vi "setpoints.vi"(6 "error in (no error)":errorcluster, 7 "setpoints":T2={"graph data interval (s)"=5.0, "sludge flow [L/s]"=0.001, "plant flow [L/s]"=0.5, "Plant Flow PID "={"proportional gain (Kc)"=10.0, "integral time (Ti, min)"=0.4, "derivative time (Td, min)"=0.0}, "Sludge PID "={"proportional gain (Kc)"=0.07, "integral time (Ti, min)"=1.0, "derivative time (Td, min)"=0.01}, "backwash"={"Filtered quality target [NTU]"=0.2, "min filtration time [s]"=3600.0, "Ripen time [s]"=600.0}, "Coagulant"={"flocculator volume (L)"=66.81, "clarifier volume (L)"=2.0, "dose updates per HRT"=10, "target clarified turbidity (NTU)"=0.6, "Coagulant mode"=enum."manual", "Coag dose [mg/L]"=5.5, "pump mL/rev"=0.255, "clarifier flow [L/s]"=0.0033, "min Coag dose [mg/L]"=2.0, "max Coag dose [mg/L]"=6.0, "Steps"=3, "HRT response delay"=2, "Ku*"=1.0, "DOM coag demand [mg/L]"=0.0, "min DOM coag demand [mg/L]"=0.0, "max DOM coag demand [mg/L]"=0.0}} {"Coagulant"."max DOM coag demand [mg/L]" min=0.0 max=20.0 step=0.1; "Coagulant"."min DOM coag demand [mg/L]" min=0.0 max=10.0 step=0.1; "Coagulant"."DOM coag demand [mg/L]" min=0.0 max=20.0 step=0.1; "Coagulant"."HRT response delay" min=1 max=10 step=1; "Coagulant"."Steps" min=3 step=1; "Coagulant"."clarifier flow [L/s]" min=0.0001 max=1.0 step=0.0001; "Coagulant"."target clarified turbidity (NTU)" min=0.1 max=5.0 step=0.01; "Coagulant"."dose updates per HRT" min=1 max=100 step=1; "Sludge PID"."derivative time (Td, min)" format="%.3f"; "Sludge PID"."integral time (Ti, min)" format="%.3f"; "Sludge PID"."proportional gain (Kc)" format="%.3f"; "Plant Flow PID"."derivative time (Td, min)" format="%.3f"; "Plant Flow PID"."integral time (Ti, min)" format="%.3f"; "Plant Flow PID"."proportional gain (Kc)" format="%.3f"; "plant flow [L/s]" min=0.05 max=1.0 step=0.05; "sludge flow [L/s]" min=0.0 max=0.05 step=0.001; "graph data interval (s)" min=1 max=1000 step=1}, 9 "ini":T1) -> (4 "error out":errorcluster, 5 "Setpoints out":T2={"graph data interval (s)"=100.0, "sludge flow [L/s]"=0.0, "plant flow [L/s]"=0.0, "Plant Flow PID "={"proportional gain (Kc)"=0.05, "integral time (Ti, min)"=1.0, "derivative time (Td, min)"=0.01}, "Sludge PID "={"proportional gain (Kc)"=0.07, "integral time (Ti, min)"=1.0, "derivative time (Td, min)"=0.01}, "backwash"={"Filtered quality target [NTU]"=0.3, "min filtration time [s]"=600.0, "Ripen time [s]"=600.0}, "Coagulant"={"flocculator volume (L)"=0.0, "clarifier volume (L)"=0.0, "dose updates per HRT"=100, "target clarified turbidity (NTU)"=0.3, "Coagulant mode"=enum."manual", "Coag dose [mg/L]"=0.0, "pump mL/rev"=0.0, "clarifier flow [L/s]"=0.5, "min Coag dose [mg/L]"=0.0, "max Coag dose [mg/L]"=0.0, "Steps"=3, "HRT response delay"=1, "Ku*"=1.0, "DOM coag demand [mg/L]"=0.0, "min DOM coag demand [mg/L]"=0.0, "max DOM coag demand [mg/L]"=0.0}} {"Coagulant"."max DOM coag demand [mg/L]" min=0.0 max=20.0 step=0.1; "Coagulant"."min DOM coag demand [mg/L]" min=0.0 max=10.0 step=0.1; "Coagulant"."DOM coag demand [mg/L]" min=0.0 max=20.0 step=0.1; "Coagulant"."HRT response delay" min=1 max=10 step=1; "Coagulant"."Steps" min=3 step=1; "Coagulant"."clarifier flow [L/s]" min=0.0001 max=1.0 step=0.0001; "Coagulant"."target clarified turbidity (NTU)" min=0.1 max=5.0 step=0.01; "Coagulant"."dose updates per HRT" min=1 max=100 step=1; "Sludge PID"."derivative time (Td, min)" format="%.3f"; "Sludge PID"."integral time (Ti, min)" format="%.3f"; "Sludge PID"."proportional gain (Kc)" format="%.3f"; "Plant Flow PID"."derivative time (Td, min)" format="%.3f"; "Plant Flow PID"."integral time (Ti, min)" format="%.3f"; "Plant Flow PID"."proportional gain (Kc)" format="%.3f"; "plant flow [L/s]" min=0.05 max=1.0 step=0.05; "sludge flow [L/s]" min=0.0 max=0.05 step=0.001; "graph data interval (s)" min=1 max=1000 step=1})   [LabVIEW 2019]
uses:
  setpoints.ctl
  backwash.ctl
  coag.ctl
  model type.ctl
  ini.ctl
  file paths.ctl
  <vilib>/Utility/config.llb/Write Key (String).vi
  <vilib>/Utility/config.llb/Read Key (String).vi
  <vilib>/Utility/config.llb/NI_LVConfig.lvlib
panel:
  out "found?":bool
  # "ramp controls"
  # "min"
  # "max"
  # "min"
  # "max"
  # "ramp controls"
  # "min"
  # "max"
  # "min"
  # "max"
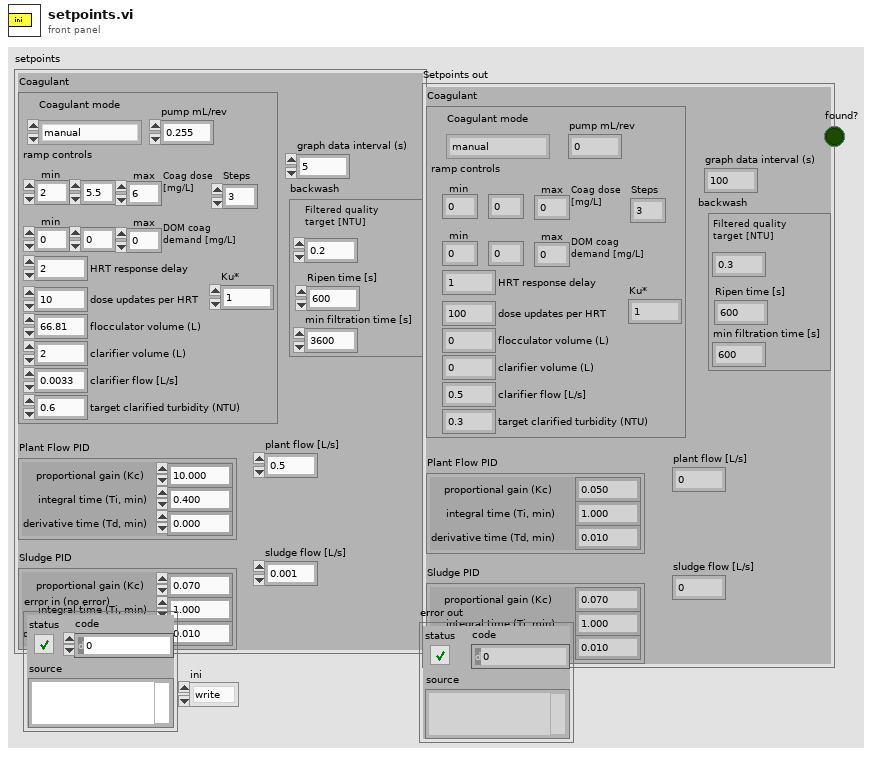
[diagram p1: front panel]
types:
  T1 = typedef "ini.ctl" = enum16{"write", "read"}
  T2 = typedef "setpoints.ctl" = cluster{"graph data interval (s)":sgl, "sludge flow [L/s]":dbl, "plant flow [L/s]":dbl, "Plant Flow PID ":cluster{"proportional gain (Kc)":dbl, "integral time (Ti, min)":dbl, "derivative time (Td, min)":dbl}, "Sludge PID ":cluster{"proportional gain (Kc)":dbl, "integral time (Ti, min)":dbl, "derivative time (Td, min)":dbl}, "backwash":T3, "Coagulant":T4}
  T3 = typedef "backwash.ctl" = cluster{"Filtered quality target [NTU]":dbl, "min filtration time [s]":dbl, "Ripen time [s]":dbl}
  T4 = typedef "coag.ctl" = cluster{"flocculator volume (L)":dbl, "clarifier volume (L)":dbl, "dose updates per HRT":u16, "target clarified turbidity (NTU)":dbl, "Coagulant mode":T5, "Coag dose [mg/L]":dbl, "pump mL/rev":dbl, "clarifier flow [L/s]":dbl, "min Coag dose [mg/L]":dbl, "max Coag dose [mg/L]":dbl, "Steps":u16, "HRT response delay":u32, "Ku*":dbl, "DOM coag demand [mg/L]":dbl, "min DOM coag demand [mg/L]":dbl, "max DOM coag demand [mg/L]":dbl}
  T5 = typedef "model type.ctl" = enum16{"manual", "ramp", "simple corrector"}
  T6 = typedef "file paths.ctl" = enum16{"read paths", "close"}
  T7 = typedef "NI_LVConfig.lvlib/Config Data RefNum.ctl" = refnum<k1>
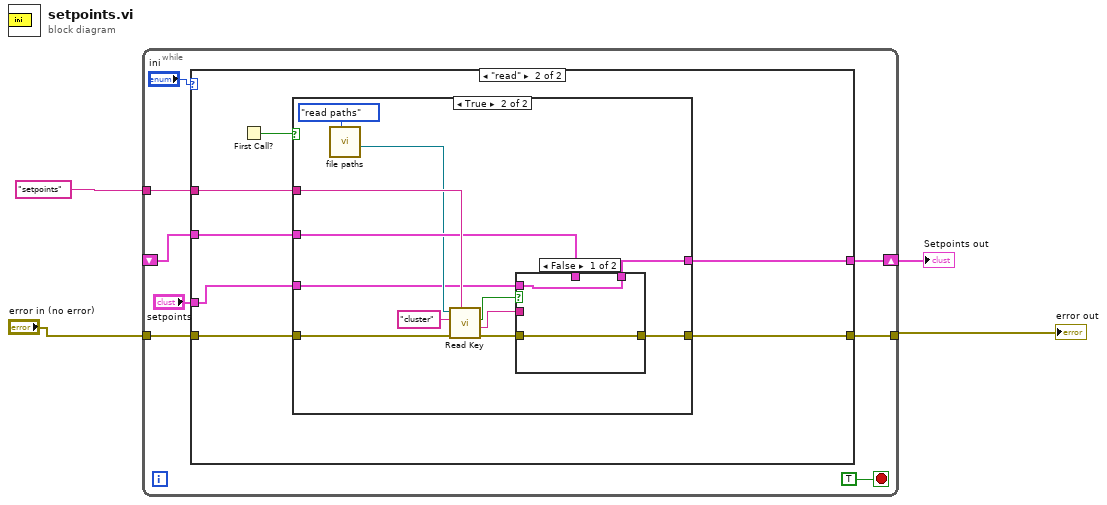
[diagram p0: block diagram]
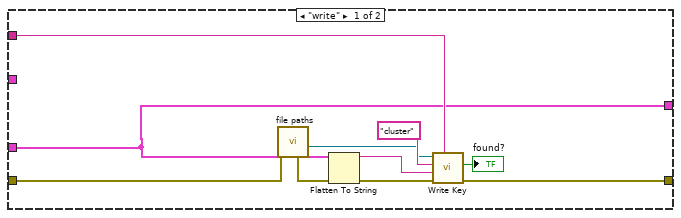
[diagram p2: hidden frame]
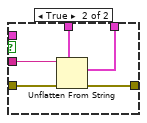
[diagram p4: hidden frame]
diagram:
  n1 = while {
    tunnel: "setpoints" ("section") -> [w10]
    tunnel: "error in (no error)" -> [w9]
    tunnel: [w8] -> w1
    shift-right: [w7] -> w3
    shift-left: _ -> [w6]
    stop <- TRUE stop-if-true
    n2 = case shown="\"read\"" "ini" {
      tunnel: w10 -> [w19 w29]
      tunnel: w9 -> [w16 w28]
      tunnel: [w18 w27] -> w8
      tunnel: w6 -> [_ w26]
      tunnel: [w13 w25] -> w7
      tunnel: "setpoints" -> [w13 w23]
      frame "write" {
        n3 = call "file paths.vi"("error in (no error)"=w16) -> ("ini"=w17:T7, "error out"=w15:errorcluster)  [unwired: 7 in, 2 out]
        n4 = Flatten To String(anything=w13, error in (no error)=w15) -> (data string=w21:string, error out=w20:errorcluster)  [unwired: 2 in, 1 out]
        n5 = call-poly <vilib>:"Write Key.vi"("section"=w19, "error in (no error)"=w20, "value"=w21, "key"="cluster", "refnum"=w17) -> ("error out"=w18:errorcluster, "found?"=→"found?":bool)  [unwired: 4 in, 1 out]
      }
      frame "read" {
        n6 = First Call?() -> (First Call?: T/F=w24:bool)
        n7 = case shown="True" w24 {
          tunnel: w29 -> [_ w40]
          tunnel: w28 -> [w31 w39]
          tunnel: [w31 w38] -> w27
          tunnel: w26 -> [w30 w37]
          tunnel: [w30 w36] -> w25
          tunnel: w23 -> [_ w32]
          frame False {
          }
          frame True {
            n8 = call "file paths.vi"("file path control"=file_paths."read paths") -> ("ini"=w35:T7)  [unwired: 7 in, 3 out]
            n9 = call-poly <vilib>:"Read Key.vi"("section"=w40, "error in (no error)"=w39, "key"="cluster", "refnum"=w35) -> ("error out"=w41:errorcluster, "value"=w42:string, "found?"=w33:bool)  [unwired: 4 in, 1 out]
            n10 = case shown="False" w33 {
              tunnel: w42 -> [_ w50]
              tunnel: w41 -> [w44 w49]
              tunnel: [w44 w48] -> w38
              tunnel: w37 -> [_ w47]
              tunnel: [w45 w46] -> w36
              tunnel: w32 -> [w45 _]
              frame False {
              }
              frame True {
                n11 = Unflatten From String(type=w47, binary string=w50, error in (no error)=w49) -> (value=w46:T2, error out=w48:errorcluster)  [unwired: 2 in, 1 out]
              }
            }
          }
        }
      }
    }
  }
  "Setpoints out" <- w3
  "error out" <- w1
